vi "Pi_Main.vi"() -> ()   [LabVIEW 2014]
uses:
  <vilib>/Analysis/4window.llb/windowTd.ctl
  <vilib>/measure/maspectr.llb/FFT Power Spectrum and PSD for 1 Chan (CDB).vi
  <vilib>/measure/NI_MAPro.lvlib
  <vilib>/Analysis/NI_AALPro.lvlib
panel:
  out "error out":errorcluster
  out "Waveform Graph":cluster{"f0":dbl, "df":dbl, "magnitude":dbl[]}(graph)
  in  "stop":bool
  out "Device Count":u32
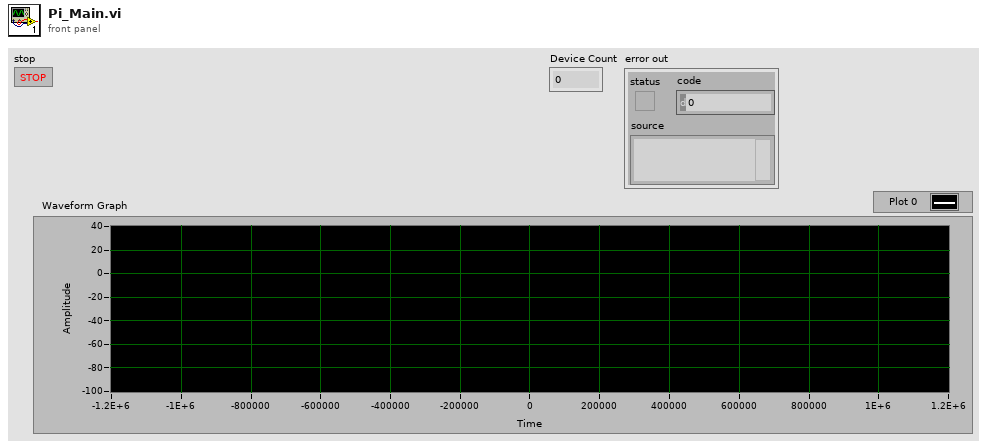
[diagram p1: front panel]
types:
  T1 = typedef "NI_AALPro.lvlib/windowTd.ctl" = u32
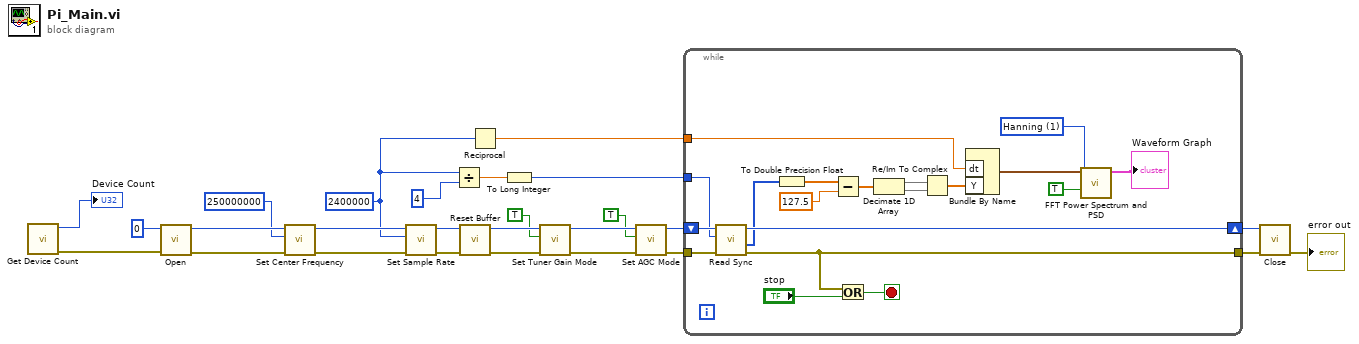
[diagram p0: block diagram]
diagram:
  w3 = u32 2400000 ("Sample Rate")
  n1 = call "Get Device Count.vi"() -> ("error out"=w25:errorcluster, "Device Count"=→"Device Count":u32)  [unwired: 10 in]
  n2 = call "Open.vi"("error in (no error)"=w25, "Device Index"=u32 0) -> ("error out"=w22:errorcluster, "DeviceRefnum Out"=w23:u64)  [unwired: 6 in]
  n3 = call "Set Center Frequency.vi"("error in (no error)"=w22, "Center Frequency"=u32 250000000, "DeviceRefnum"=w23) -> ("error out"=w20:errorcluster, "DeviceRefnum Out"=w19:u64)  [unwired: 6 in, 1 out]
  n4 = call "Set Sample Rate.vi"("error in (no error)"=w20, "Sample Rate"=w3, "DeviceRefnum"=w19) -> ("error out"=w17:errorcluster, "DeviceRefnum Out"=w18:u64)  [unwired: 6 in, 1 out]
  n5 = Divide(x=w3, y=u32 4) -> (x/y=w2:dbl)
  n6 = call "Reset Buffer.vi"("error in (no error)"=w17, "DeviceRefnum"=w18) -> ("error out"=w15:errorcluster, "DeviceRefnum Out"=w16:u64)  [unwired: 7 in, 1 out]
  n7 = Reciprocal(x=w3) -> (1/x=w5:dbl)
  n8 = To Long Integer(number=w2) -> (32bit integer=w1:i32)
  n9 = call "Set Tuner Gain Mode.vi"("error in (no error)"=w15, "AutoGain"=TRUE, "DeviceRefnum"=w16) -> ("error out"=w13:errorcluster, "DeviceRefnum Out"=w12:u64)  [unwired: 6 in, 1 out]
  n10 = call "Set AGC Mode.vi"("error in (no error)"=w13, "AGC Enable"=TRUE, "DeviceRefnum"=w12) -> ("error out"=w10:errorcluster, "DeviceRefnum Out"=w9:u64)  [unwired: 6 in, 1 out]
  n11 = while {
    tunnel: w10 -> [w45]
    shift-right: [w43] -> w8
    shift-left: w9 -> [w44]
    tunnel: [w42] -> w7
    tunnel: w5 -> [w33]
    tunnel: w1 -> [w28]
    stop <- w40 stop-if-true
    w31 = T1 1 items=["Rectangle"=0, "Hanning"=1, "Hamming"=2, "Blackman-Harris"=3, "Exact Blackman"=4, "Blackman"=5, "Flat Top"=6, "4 Term B-Harris "=7, "7 Term B-Harris"=8, "Low Sidelobe"=9, "Blackman Nuttall"=11, "Triangle"=30, "Bartlett-Hanning"=31, "Bohman"=32, "Parzen"=33, "Welch"=34, "Kaiser"=60, "Dolph-Chebyshev"=61, "Gaussian"=62] ("window")
    n12 = call "Read Sync.vi"("error in (no error)"=w45, "Number Of Samples"=w28, "DeviceRefnum"=w44) -> ("error out"=w42:errorcluster, "Sample Buffer"=w27:u8[], "DeviceRefnum Out"=w43:u64)  [unwired: 5 in, 1 out]
    n13 = To Double Precision Float(number=w27) -> (double precision float=w39:dbl[])
    n14 = Subtract(x=w39, y=127.5) -> (x-y=w38:dbl[])
    n15 = Or(x=w42, y="stop") -> (x .or. y?=w40:bool)
    n16 = Decimate 1D Array(w38) -> (w37:dbl[], w36:dbl[])
    n17 = Re/Im To Complex(1:w36, 2:w37) -> (0:w34:cdb[])
    n18 = Bundle By Name("dt"=w33, "Y"=w34) -> (w32:waveform(cdb))  [unwired: 1 in]
    n19 = call-poly <vilib>:"FFT Power Spectrum and PSD.vi"("dB On (F)"=TRUE, "window"=w31, "time signal"=w32) -> ("Power Spectrum / PSD"=→"Waveform Graph":cluster{"f0":dbl, "df":dbl, "magnitude":dbl[]})  [unwired: 5 in, 3 out]
  }
  n20 = call "Close.vi"("error in (no error)"=w7, "DeviceRefnum"=w8) -> ("error out"=→"error out":errorcluster)  [unwired: 8 in, 1 out]
